vi "Initialize.vi"(8 "error in (no error)":errorcluster, 11 "Sonicator Module State Cluster":T1={"State"=enum."Idle", "Start Time"=timestamp(0 s since 1904-01-01), "Current Time"=timestamp(0 s since 1904-01-01), "Sonicator Module Config"={"GUID"="", "Drop Coords"={"Horizontal"=0, "Vertical"=0}, "Process Name"="", "User name"="", "Queue Name"="", "Settings"={"Cycle Period"=500.0, "Sonicator Type"="Sonic Systems P100", "SS P100 Settings"={"VISA resource name"="", "Simulated?"=FALSE}, "Setpoint (µm)"=0.0, "Cutoff (W)"=0.0}, "Load Count"=0}, "Output Error"=FALSE, "Log Started"=FALSE, "First Iteration"=FALSE, "Data"={"Sonicator Amp Value"=0.0, "Sonicator Power Value"=0.0}, "Sonicator On?"=enum."Off"}) -> (0 "error out":errorcluster, 1 "Initialized":bool, 3 "Sonicator Module State Cluster":T1={"State"=enum."Idle", "Start Time"=timestamp(0 s since 1904-01-01), "Current Time"=timestamp(0 s since 1904-01-01), "Sonicator Module Config"={"GUID"="", "Drop Coords"={"Horizontal"=0, "Vertical"=0}, "Process Name"="", "User name"="", "Queue Name"="", "Settings"={"Cycle Period"=500.0, "Sonicator Type"="Sonic Systems P100", "SS P100 Settings"={"VISA resource name"="", "Simulated?"=FALSE}, "Setpoint (µm)"=0.0, "Cutoff (W)"=0.0}, "Load Count"=0}, "Output Error"=FALSE, "Log Started"=FALSE, "First Iteration"=FALSE, "Data"={"Sonicator Amp Value"=0.0, "Sonicator Power Value"=0.0}, "Sonicator On?"=enum."Off"})   [LabVIEW 2018, in "Sonicator Module.lvlib" / "Sonicator Module Engine.lvlib"]
uses:
  Sonicator Module Engine.lvlib
  Feed Module/Controls/Sonicator Module State Cluster.ctl
  Pump Module Folder/Measure Instrument/State Enum.ctl
  Feed Module/Controls/Sonicator Module Config Cluster.ctl
  <vilib>/Utility/miscctls.llb/LVPoint32TypeDef.ctl
  Feed Module/Controls/Sonicator Module Settings Cluster.ctl
  Sonic Systems P100/Sonic Systems P100 Settings.ctl
  Tag VIs/Tag FGV Operation Enum.ctl
  Shared Variables/Dynamic Shared Variables.lvlib
  Sonic Systems P100/Sonic Systems P100.lvlib
  Sonicator Module.lvlib
  Pump Module Folder/Measure Instrument/Pump Module Engine.lvlib
panel:
  # "Sonicator Settings"
  # "Sonicator Settings"
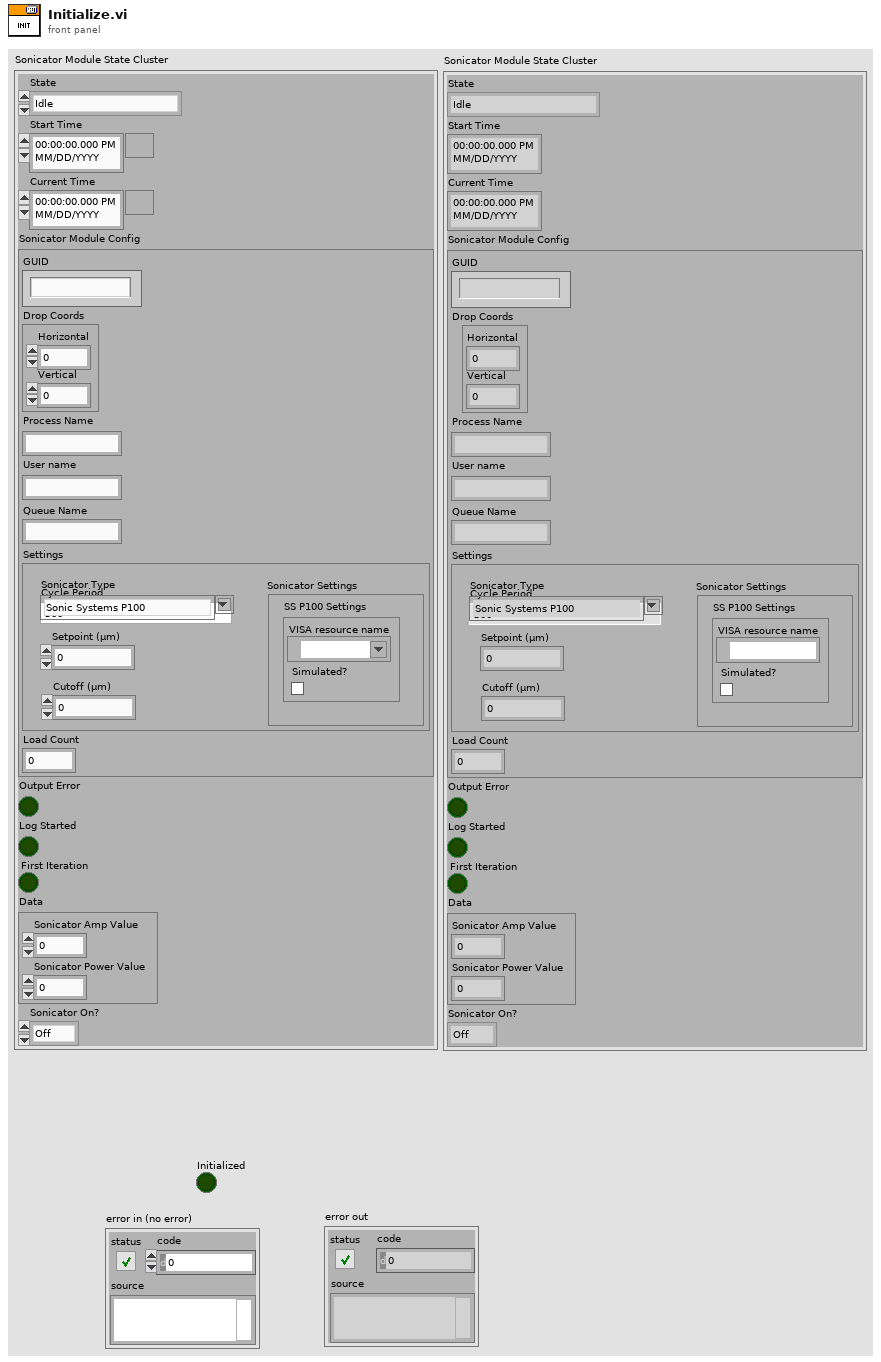
[diagram p1: front panel]
types:
  T1 = typedef "Sonicator Module.lvlib/Sonicator Module State Cluster.ctl" = cluster{"State":T2, "Start Time":timestamp, "Current Time":timestamp, "Sonicator Module Config":T3, "Output Error":bool, "Log Started":bool, "First Iteration":bool, "Data":cluster{"Sonicator Amp Value":dbl, "Sonicator Power Value":dbl}, "Sonicator On?":enum16{"Off", "On", "Not Initialized", "Over Cutoff"}}
  T2 = typedef "Pump Module.lvlib/Pump Module Engine.lvlib/State Enum.ctl" = enum16{"Measuring", "Idle", "Paused"}
  T3 = typedef "Sonicator Module.lvlib/Sonicator Module Config Cluster.ctl" = cluster{"GUID":string, "Drop Coords":T4, "Process Name":string, "User name":string, "Queue Name":string, "Settings":T5, "Load Count":i32}
  T4 = typedef "LVPoint32TypeDef.ctl" = cluster{"Horizontal":i32, "Vertical":i32}
  T5 = typedef "Sonicator Module.lvlib/Sonicator Module Settings Cluster.ctl" = cluster{"Cycle Period":dbl, "Sonicator Type":string, "SS P100 Settings":T6, "Setpoint (µm)":dbl, "Cutoff (W)":dbl}
  T6 = typedef "Sonic Systems P100.lvlib/Sonic Systems P100 Settings.ctl" = cluster{"VISA resource name":refnum<visa-resource-name>, "Simulated?":bool}
  T7 = typedef "Tag FGV Operation Enum.ctl" = enum16{"Init", "Set Notification Queue", "Create Tag", "Commit", "Write Tag (Numeric)", "Write Tag (Boolean)", "Read All Tags", "Read One Tag", "Delete Tag Category", "Set Alarm Parameters (Numeric)", "Set Alarm Parameters (Boolean)", "Enable All Alarms", "Disable All Alarms", "Delete All Tags", "Read Alarms", "Ack Alarm", "Read Alarm Parameters (Numeric)", "Read Alarm Parameters (Boolean)"}
  T8 = cluster{"Amplitude Tag":string, "Power Tag":string, "Output Device Tag":string}
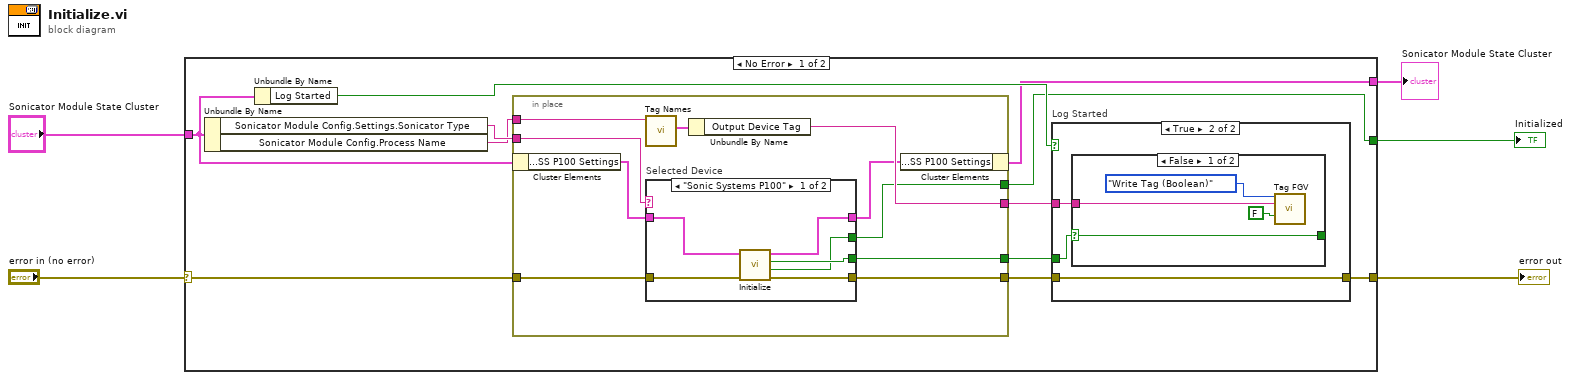
[diagram p0: block diagram]
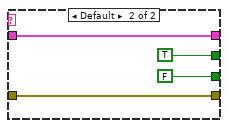
[diagram p2: hidden frame]
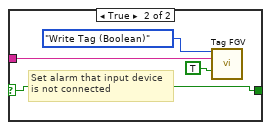
[diagram p4: hidden frame]
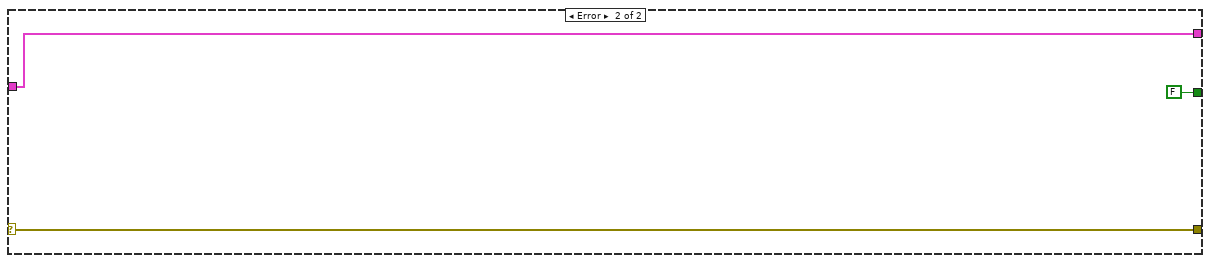
[diagram p5: hidden frame]
diagram:
  n1 = case shown="No Error" "error in (no error)" {
    selector: "error in (no error)" -> [w15 w51]
    tunnel: [w12 w51] -> w4
    tunnel: "Sonicator Module State Cluster" -> [w9 w50]
    tunnel: [w8 w50] -> w1
    tunnel: [w6 FALSE ("Initialized")] -> w3
    frame No Error {
      n2 = Unbundle By Name(w9) -> ("Sonicator Module Config.Settings.Sonicator Type"=w16:string, "Sonicator Module Config.Process Name"=w14:string)
      n3 = Unbundle By Name(w9) -> ("Log Started"=w10:bool)
      n4 = in-place {
        in-place-border: w16 -> [w26]
        in-place-border: w15 -> [w25]
        in-place-border: w14 -> [w24]
        in-place-border: [w23] -> w13
        in-place-border: [w21] -> w11
        in-place-border: [w18] -> w7
        in-place-border: [w17] -> w6
        n5 = in-place-cluster #1(w9) -> ("Sonicator Module Config.Settings.SS P100 Settings"=w20:T6)
        n6 = call "Tag Names.vi"("Process Name"=w24) -> ("SC Tags"=w22:T8)  [unwired: 8 in, 2 out]
        n7 = case "Selected Device" shown="\"Sonic Systems P100\"" w26 {
          tunnel: w20 -> [w32 w36]
          tunnel: w25 -> [w31 w35]
          tunnel: [w29 w35] -> w23
          tunnel: [w30 w36] -> w19
          tunnel: [w28 FALSE ("Connection Error")] -> w18
          tunnel: [w27 TRUE ("Initialized")] -> w17
          frame "Sonic Systems P100" {
            n8 = call "Initialize.vi"("error in (no error)"=w31, "SS P100 Settings"=w32) -> ("error out"=w29:errorcluster, "Initialized"=w27:bool, "Connection Error"=w28:bool, "SS P100 Settings"=w30:T6)  [unwired: 6 in]
          }
          frame Default {
          }
        }
        n9 = Unbundle By Name(w22) -> ("Output Device Tag"=w21:string)
        n10 = in-place-cluster #1("Sonicator Module Config.Settings.SS P100 Settings"=w19) -> (w8:T1)
      }
      n11 = case "Log Started" shown="True" w10 {
        tunnel: w13 -> [w37 w38]
        tunnel: [w37 w38] -> w12
        tunnel: w11 -> [_ w40]
        tunnel: w7 -> [_ w39]
        frame False {
        }
        frame True {
          n12 = case shown="False" w39 {
            selector: w39 -> [w44 w48]
            tunnel: [w44 w48] -> _
            tunnel: w40 -> [w42 w46]
            frame False {
              n13 = call "Tag FGV.vi"("Operation"=Tag_FGV_Operation_Enum."Write Tag (Boolean)", "Tag Name"=w42, "Data"=FALSE) -> ()  [unwired: 5 in, 8 out]
            }
            frame True {
              # "Set alarm that input device\nis not connected"
              n14 = call "Tag FGV.vi"("Operation"=Tag_FGV_Operation_Enum."Write Tag (Boolean)", "Tag Name"=w46, "Data"=TRUE) -> ()  [unwired: 5 in, 8 out]
            }
          }
        }
      }
    }
    frame Error {
    }
  }
  "error out" <- w4
  "Initialized" <- w3
  "Sonicator Module State Cluster" <- w1
